vi "ROI_calculate_embryo_ROIs.vi"(0 "Angle":dbl, 1 "b":dbl, 2 "Embryo's ends":dbl[][](array[numeric]), 3 "Slope a":dbl, 4 "XY positions":dbl[][](array[numeric])) -> (5 "ROIs":dbl[][](array[numeric]))   [LabVIEW 2015]
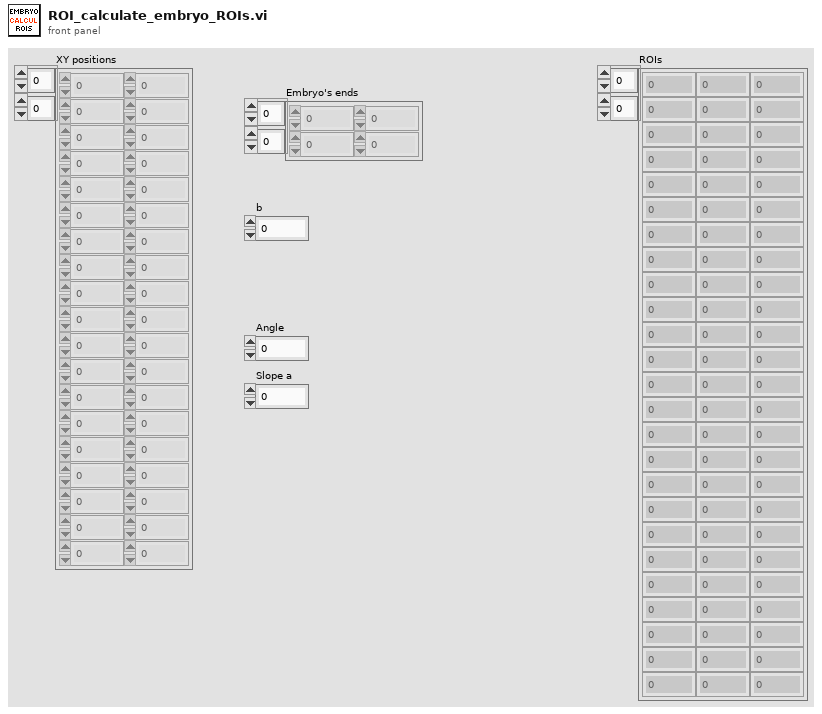
[diagram p1: front panel]
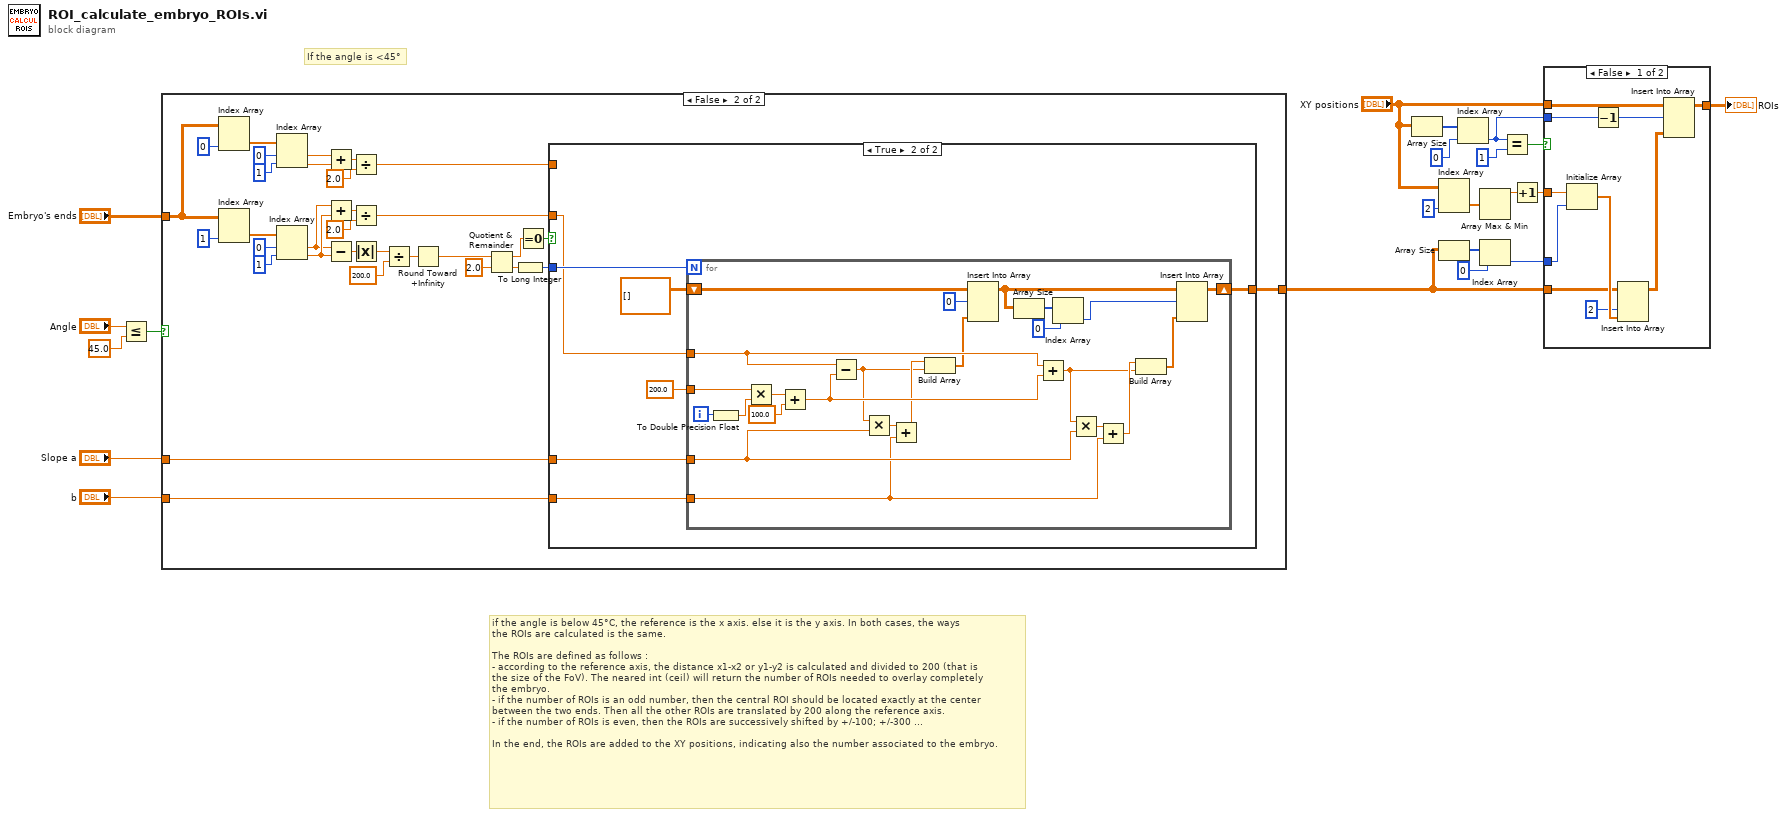
[diagram p0: block diagram]
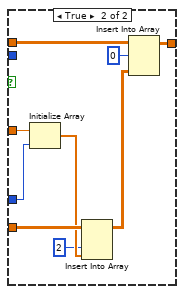
[diagram p2: hidden frame]
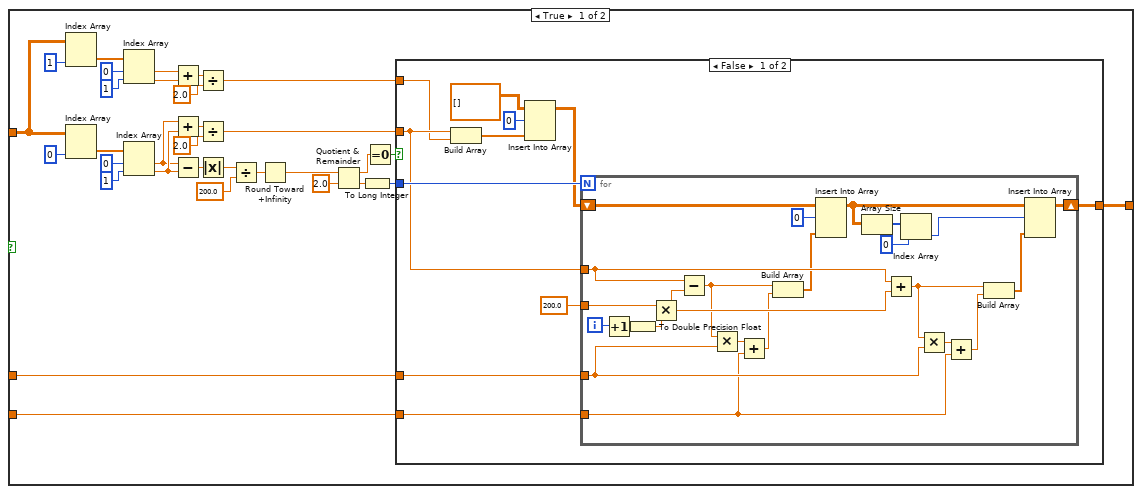
[diagram p3: hidden frame]
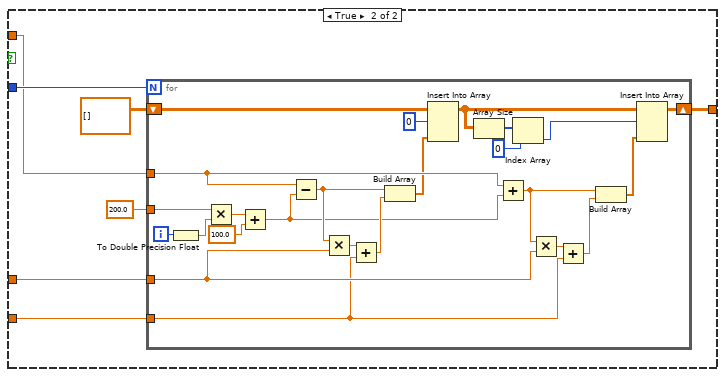
[diagram p4: hidden frame]
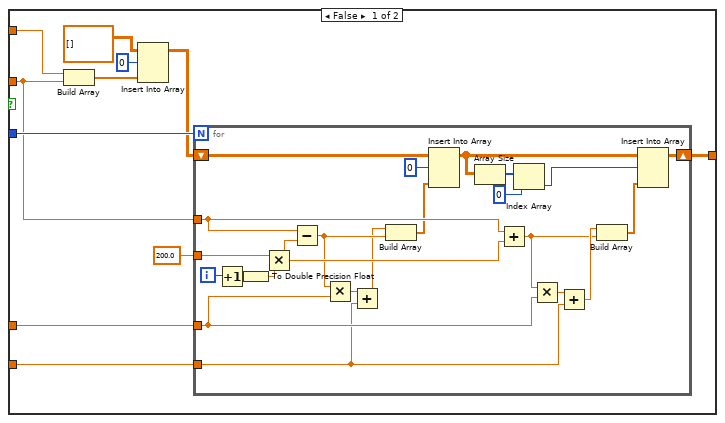
[diagram p5: hidden frame]
diagram:
  # "if the angle is below 45°C, the reference is the x axis. else it is the y axis. In both cases, the ways\nthe ROIs are calculated is the same.\n\nThe ROIs are defined as follows :\n- according to the reference axis, the distance x1-x2 or y1-y2 is calculated and divided to 200 (that is\nthe size of the FoV). The neared int (ceil) will return the number of ROIs needed to overlay completely\nthe embryo.\n- if the number of ROIs is an odd number, then the central ROI should be located exactly at the center between the two ends. Then all the other ROIs are translated by 200 along the reference axis.\n- if the number of ROIs is even, then the ROIs are successively shifted by +/-100; +/-300 ... \n\nIn the end, the ROIs are added to the XY positions, indicating also the number associated to the embryo."
  # "If the angle is <45°"
  n1 = Less Or Equal?(x="Angle", y=45.0) -> (x <= y?=w12:bool)
  n2 = case shown="False" w12 {
    tunnel: "Embryo's ends" -> [w43 w140]
    tunnel: "Slope a" -> [w32 w129]
    tunnel: "b" -> [w31 w128]
    tunnel: [w30 w127] -> w3
    frame True {
      n3 = Index Array(array=w43, index (col)=1 ("disabled index (col)")) -> (element=w39:dbl[])  [unwired: 1 in]
      n4 = Index Array(array=w43, index (col)=0 ("disabled index (col)")) -> (element=w52:dbl[])  [unwired: 1 in]
      n5 = Index Array(array=w39, index #1=0 ("index"), index #2=1 ("index")) -> (element #1=w38:dbl, element #2=w37:dbl)
      n6 = Index Array(array=w52, index #1=0 ("index"), index #2=1 ("index")) -> (element #1=w44:dbl, element #2=w45:dbl)
      n7 = Add(x=w38, y=w37) -> (x+y=w28:dbl)
      n8 = Add(x=w44, y=w45) -> (x+y=w29:dbl)
      n9 = Subtract(x=w44, y=w45) -> (x-y=w49:dbl)
      n10 = Divide(x=w28, y=2.0 ("x")) -> (x/y=w36:dbl)
      n11 = Divide(x=w29, y=2.0 ("x")) -> (x/y=w35:dbl)
      n12 = Absolute Value(x=w49) -> (abs(x)=w25:dbl)
      n13 = Divide(x=w25, y=200.0) -> (x/y=w23:dbl)
      n14 = Round Toward +Infinity(x=w23) -> (ceil(x): smallest int >= x=w22:dbl)
      n15 = Quotient & Remainder(x=w22, y=2.0) -> (x-y*floor(x/y)=w47:dbl, floor(x/y)=w34:dbl)
      n16 = To Long Integer(number=w34) -> (32bit integer=w33:i32)
      n17 = Equal To 0?(x=w47) -> (x = 0?=w46:bool)
      n18 = case shown="False" w46 {
        tunnel: w36 -> [w56 _]
        tunnel: w35 -> [w57 w89]
        tunnel: w33 -> [w64 w94]
        tunnel: w32 -> [w62 w92]
        tunnel: w31 -> [w61 w91]
        tunnel: [w60 w90] -> w30
        frame False {
          n19 = Build Array(w57, w56) -> (w55:dbl[])
          n20 = Insert Into Array(array=dbl[][] [] ("appended array"), index (row)=0, new element=w55) -> (w54:dbl[][])  [unwired: 1 in]
          n21 = for {
            N: w64 -> [_]
            tunnel: w57 -> [w81]
            shift-right: [w70] -> w60
            shift-left: w54 -> [w73]
            tunnel: 200.0 ("y") -> [w86]
            tunnel: w62 -> [w79]
            tunnel: w61 -> [w78]
            i -> [w87]
            n22 = Increment(x=w87) -> (x+1=w85:i32)
            n23 = To Double Precision Float(number=w85) -> (double precision float=w84:dbl)
            n24 = Multiply(x=w86, y=w84) -> (x*y=w80:dbl)
            n25 = Subtract(x=w81, y=w80) -> (x-y=w76:dbl)
            n26 = Multiply(x=w76, y=w79) -> (x*y=w83:dbl)
            n27 = Add(x=w83, y=w78) -> (x+y=w77:dbl)
            n28 = Build Array(w76, w77) -> (w71:dbl[])
            n29 = Insert Into Array(array=w73, index (row)=0, new element=w71) -> (w68:dbl[][])  [unwired: 1 in]
            n30 = Array Size(array=w68) -> (size(s)=w67:i32[])
            n31 = Add(x=w81, y=w80) -> (x+y=w75:dbl)
            n32 = Index Array(array=w67, index=0) -> (element=w65:i32)
            n33 = Multiply(x=w75, y=w79) -> (x*y=w82:dbl)
            n34 = Add(x=w82, y=w78) -> (x+y=w74:dbl)
            n35 = Build Array(w75, w74) -> (w69:dbl[])
            n36 = Insert Into Array(array=w68, index (row)=w65, new element=w69) -> (w70:dbl[][])  [unwired: 1 in]
          }
        }
        frame True {
          n37 = for {
            N: w94 -> [_]
            tunnel: w89 -> [w116]
            shift-right: [w106] -> w90
            shift-left: dbl[][] [] ("appended array") -> [w109]
            tunnel: 200.0 ("y") -> [w99]
            tunnel: w92 -> [w115]
            tunnel: w91 -> [w114]
            i -> [w100]
            n38 = To Double Precision Float(number=w100) -> (double precision float=w98:dbl)
            n39 = Multiply(x=w99, y=w98) -> (x*y=w97:dbl)
            n40 = Add(x=w97, y=100.0) -> (x+y=w95:dbl)
            n41 = Subtract(x=w116, y=w95) -> (x-y=w112:dbl)
            n42 = Multiply(x=w112, y=w115) -> (x*y=w118:dbl)
            n43 = Add(x=w118, y=w114) -> (x+y=w113:dbl)
            n44 = Build Array(w112, w113) -> (w107:dbl[])
            n45 = Insert Into Array(array=w109, index (row)=0, new element=w107) -> (w104:dbl[][])  [unwired: 1 in]
            n46 = Array Size(array=w104) -> (size(s)=w103:i32[])
            n47 = Add(x=w116, y=w95) -> (x+y=w111:dbl)
            n48 = Index Array(array=w103, index=0) -> (element=w101:i32)
            n49 = Multiply(x=w111, y=w115) -> (x*y=w117:dbl)
            n50 = Add(x=w117, y=w114) -> (x+y=w110:dbl)
            n51 = Build Array(w111, w110) -> (w105:dbl[])
            n52 = Insert Into Array(array=w104, index (row)=w101, new element=w105) -> (w106:dbl[][])  [unwired: 1 in]
          }
        }
      }
    }
    frame False {
      n53 = Index Array(array=w140, index (col)=0 ("disabled index (col)")) -> (element=w136:dbl[])  [unwired: 1 in]
      n54 = Index Array(array=w140, index (col)=1 ("disabled index (col)")) -> (element=w149:dbl[])  [unwired: 1 in]
      n55 = Index Array(array=w136, index #1=0 ("index"), index #2=1 ("index")) -> (element #1=w135:dbl, element #2=w134:dbl)
      n56 = Index Array(array=w149, index #1=0 ("index"), index #2=1 ("index")) -> (element #1=w141:dbl, element #2=w142:dbl)
      n57 = Add(x=w135, y=w134) -> (x+y=w125:dbl)
      n58 = Add(x=w141, y=w142) -> (x+y=w126:dbl)
      n59 = Subtract(x=w141, y=w142) -> (x-y=w146:dbl)
      n60 = Divide(x=w125, y=2.0 ("x")) -> (x/y=w133:dbl)
      n61 = Divide(x=w126, y=2.0 ("x")) -> (x/y=w132:dbl)
      n62 = Absolute Value(x=w146) -> (abs(x)=w122:dbl)
      n63 = Divide(x=w122, y=200.0) -> (x/y=w120:dbl)
      n64 = Round Toward +Infinity(x=w120) -> (ceil(x): smallest int >= x=w119:dbl)
      n65 = Quotient & Remainder(x=w119, y=2.0) -> (x-y*floor(x/y)=w144:dbl, floor(x/y)=w131:dbl)
      n66 = To Long Integer(number=w131) -> (32bit integer=w130:i32)
      n67 = Equal To 0?(x=w144) -> (x = 0?=w143:bool)
      n68 = case shown="True" w143 {
        tunnel: w133 -> [w152 _]
        tunnel: w132 -> [w151 w186]
        tunnel: w130 -> [w161 w191]
        tunnel: w129 -> [w159 w189]
        tunnel: w128 -> [w158 w188]
        tunnel: [w157 w187] -> w127
        frame False {
          n69 = Build Array(w152, w151) -> (w154:dbl[])
          n70 = Insert Into Array(array=dbl[][] [] ("appended array"), index (row)=0, new element=w154) -> (w153:dbl[][])  [unwired: 1 in]
          n71 = for {
            N: w161 -> [_]
            tunnel: w151 -> [w178]
            shift-right: [w171] -> w157
            shift-left: w153 -> [w174]
            tunnel: 200.0 ("y") -> [w183]
            tunnel: w159 -> [w176]
            tunnel: w158 -> [w175]
            i -> [w184]
            n72 = Increment(x=w184) -> (x+1=w182:i32)
            n73 = To Double Precision Float(number=w182) -> (double precision float=w181:dbl)
            n74 = Multiply(x=w183, y=w181) -> (x*y=w177:dbl)
            n75 = Subtract(x=w178, y=w177) -> (x-y=w165:dbl)
            n76 = Multiply(x=w165, y=w176) -> (x*y=w180:dbl)
            n77 = Add(x=w180, y=w175) -> (x+y=w164:dbl)
            n78 = Build Array(w164, w165) -> (w172:dbl[])
            n79 = Insert Into Array(array=w174, index (row)=0, new element=w172) -> (w169:dbl[][])  [unwired: 1 in]
            n80 = Array Size(array=w169) -> (size(s)=w168:i32[])
            n81 = Add(x=w178, y=w177) -> (x+y=w162:dbl)
            n82 = Index Array(array=w168, index=0) -> (element=w166:i32)
            n83 = Multiply(x=w162, y=w176) -> (x*y=w179:dbl)
            n84 = Add(x=w179, y=w175) -> (x+y=w163:dbl)
            n85 = Build Array(w163, w162) -> (w170:dbl[])
            n86 = Insert Into Array(array=w169, index (row)=w166, new element=w170) -> (w171:dbl[][])  [unwired: 1 in]
          }
        }
        frame True {
          n87 = for {
            N: w191 -> [_]
            tunnel: w186 -> [w213]
            shift-right: [w207] -> w187
            shift-left: dbl[][] [] ("appended array") -> [w210]
            tunnel: 200.0 ("y") -> [w200]
            tunnel: w189 -> [w212]
            tunnel: w188 -> [w211]
            i -> [w201]
            n88 = To Double Precision Float(number=w201) -> (double precision float=w199:dbl)
            n89 = Multiply(x=w200, y=w199) -> (x*y=w198:dbl)
            n90 = Add(x=w198, y=100.0) -> (x+y=w196:dbl)
            n91 = Subtract(x=w213, y=w196) -> (x-y=w194:dbl)
            n92 = Multiply(x=w194, y=w212) -> (x*y=w215:dbl)
            n93 = Add(x=w215, y=w211) -> (x+y=w195:dbl)
            n94 = Build Array(w195, w194) -> (w208:dbl[])
            n95 = Insert Into Array(array=w210, index (row)=0, new element=w208) -> (w205:dbl[][])  [unwired: 1 in]
            n96 = Array Size(array=w205) -> (size(s)=w204:i32[])
            n97 = Add(x=w213, y=w196) -> (x+y=w192:dbl)
            n98 = Index Array(array=w204, index=0) -> (element=w202:i32)
            n99 = Multiply(x=w192, y=w212) -> (x*y=w214:dbl)
            n100 = Add(x=w214, y=w211) -> (x+y=w193:dbl)
            n101 = Build Array(w193, w192) -> (w206:dbl[])
            n102 = Insert Into Array(array=w205, index (row)=w202, new element=w206) -> (w207:dbl[][])  [unwired: 1 in]
          }
        }
      }
    }
  }
  n103 = Array Size(array="XY positions") -> (size(s)=w21:i32[])
  n104 = Index Array(array="XY positions", index (col)=2 ("disabled index (col)")) -> (element=w7:dbl[])  [unwired: 1 in]
  n105 = Array Size(array=w3) -> (size(s)=w1:i32[])
  n106 = Index Array(array=w21, index=0) -> (element=w16:i32)
  n107 = Array Max & Min(array=w7) -> (max value=w6:dbl)  [unwired: 3 out]
  n108 = Index Array(array=w1, index=0) -> (element=w2:i32)
  n109 = Equal?(x=w16, y=1) -> (x = y?=w18:bool)
  n110 = Increment(x=w6) -> (x+1=w5:dbl)
  n111 = case shown="False" w18 {
    tunnel: "XY positions" -> [w225 w234]
    tunnel: [w223 w232] -> w17
    tunnel: w16 -> [w224 _]
    tunnel: w3 -> [w217 w229]
    tunnel: w5 -> [w219 w231]
    tunnel: w2 -> [w218 w230]
    frame False {
      n112 = Initialize Array(w219, w218) -> (w221:dbl[])
      n113 = Decrement(x=w224) -> (x-1=w222:i32)
      n114 = Insert Into Array(array=w217, index (col)=2 ("disabled index (col)"), new element=w221) -> (w216:dbl[][])  [unwired: 1 in]
      n115 = Insert Into Array(array=w225, index (row)=w222, new element=w216) -> (w223:dbl[][])  [unwired: 1 in]
    }
    frame True {
      n116 = Initialize Array(w231, w230) -> (w228:dbl[])
      n117 = Insert Into Array(array=w229, index (col)=2 ("disabled index (col)"), new element=w228) -> (w226:dbl[][])  [unwired: 1 in]
      n118 = Insert Into Array(array=w234, index (row)=0, new element=w226) -> (w232:dbl[][])  [unwired: 1 in]
    }
  }
  "ROIs" <- w17
